vi "Convert to Absolute Path.vi"(11 "System Definition File":path) -> (3 "Absolute Path":path)   [LabVIEW 2019, in "Scan Engine Example Support.lvlib"]
uses:
  Scan Engine Example Support.lvlib
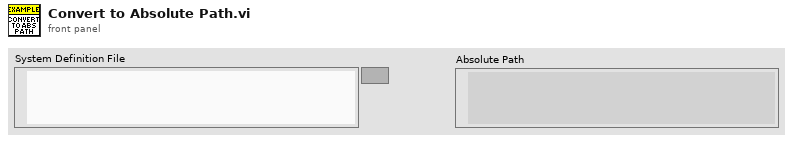
[diagram p1: front panel]
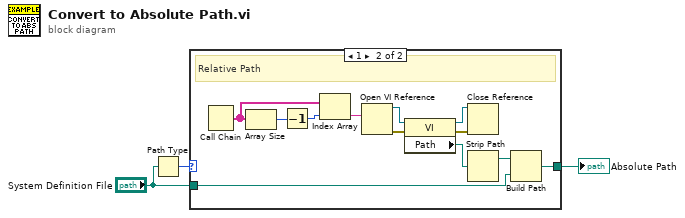
[diagram p0: block diagram]
diagram:
  n1 = Path Type(1:"System Definition File") -> (0:w1:i16)
  n2 = case shown="1" w1 {
    tunnel: "System Definition File" -> [w4 w16]
    tunnel: [w4 w15] -> w3
    frame 0, Default {
      # "Absolute Path or Not A Path"
    }
    frame 1 {
      # "Relative Path"
      n3 = Call Chain() -> (call chain=w11:string[])
      n4 = Array Size(array=w11) -> (size(s)=w12:i32)
      n5 = Decrement(x=w12) -> (x-1=w13:i32)
      n6 = Index Array(array=w11, index=w13) -> (element=w10:string)
      n7 = Open VI Reference(vi path=w10) -> (vi reference=w9:refnum<vi>, error out=w7:errorcluster)  [unwired: 5 in]
      n8 = property class="VI"(reference=w9, error in=w7) -> (reference out=w8:refnum<vi>, error out=w6:errorcluster, "Path"=w5:path)
      n9 = Close Reference(reference=w8, error in (no error)=w6) -> ()  [unwired: 1 out]
      n10 = Strip Path(path=w5) -> (stripped path=w14:path)  [unwired: 1 out]
      n11 = Build Path(base path=w14, name or relative path=w16) -> (appended path=w15:path)
    }
  }
  "Absolute Path" <- w3
